vi "ApplyPasswords.vi"() -> ()   [LabVIEW 2009]
panel:
  in  "New Description":string
  in  "Cancel":bool
  in  "Apply":bool
  out "Project Name":string
  in  "Replace Description?":bool=TRUE
  in  "Clear History?":bool=TRUE
  in  "New Password (if empty unlocked)":string
  in  "Old Passwords":string[](array[string])
  out "Progress":dbl(slide) scale=0.0..1.0
  out "Processing VI Name":string
  out "error out":errorcluster
  # "Apply Passwords To Project VIs"
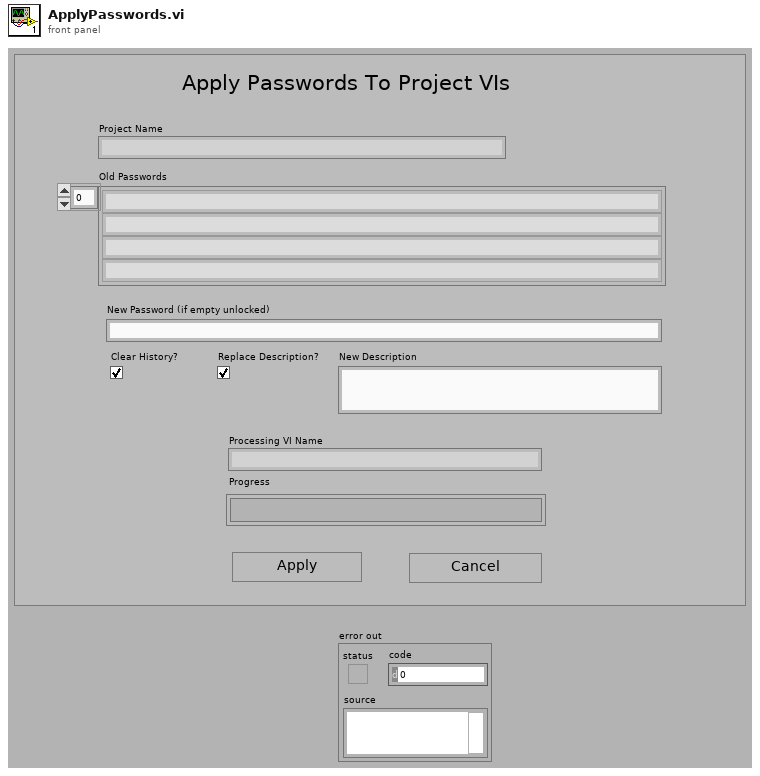
[diagram p1: front panel]
types:
  T1 = enum8{"Enabled", "Disabled", "Disabled and Grayed Out"}
  T2 = enum32{"invalid lock state", "Not Locked", "Locked (No Password)", "Password-protected"}
  T3 = enum32{"invalid VI type", "Standard VI", "Control VI", "Global VI", "Polymorphic VI", "Configuration VI", "SubSystem", "Facade VI", "Method VI", "Statechart Diagram VI"}
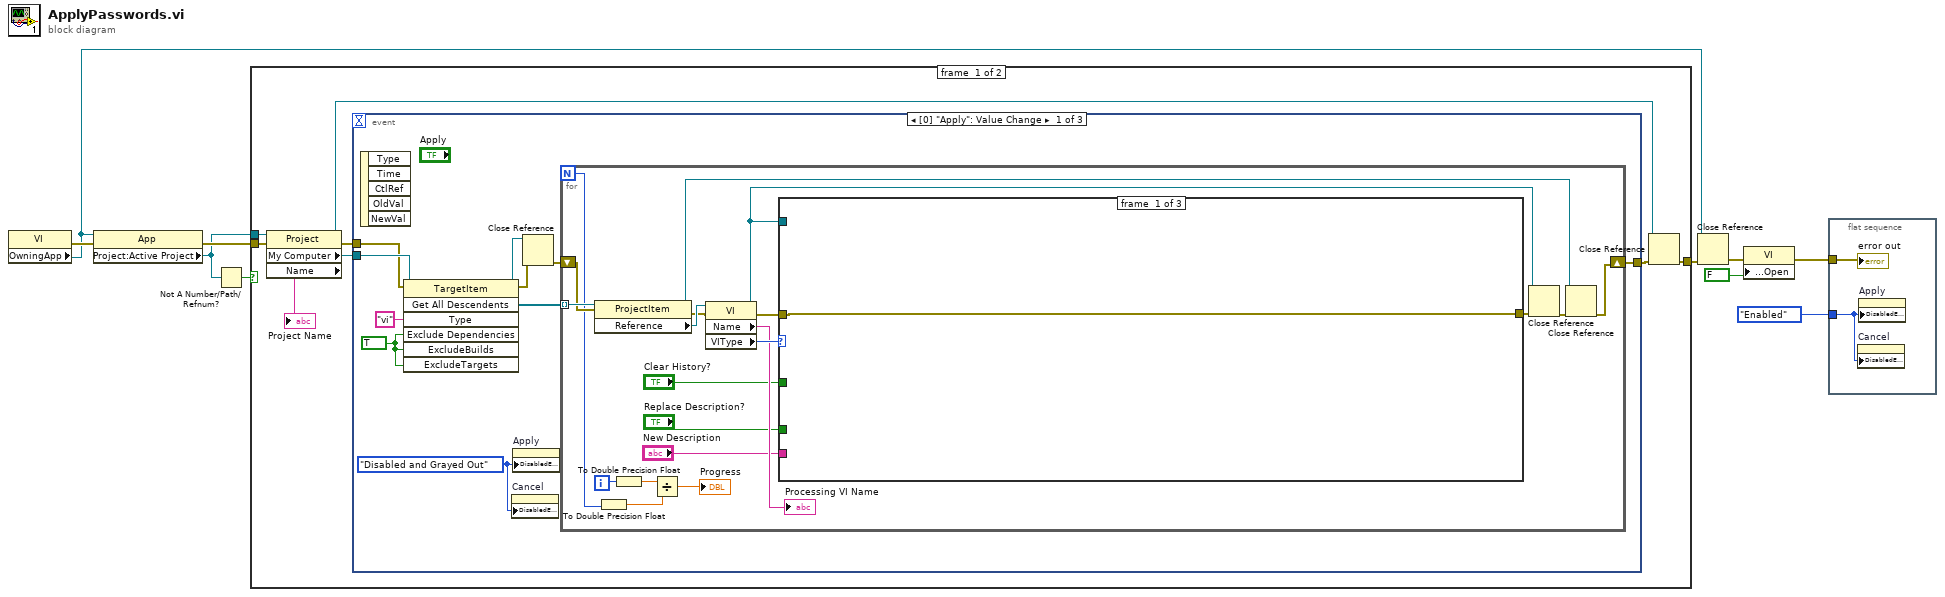
[diagram p0: block diagram]
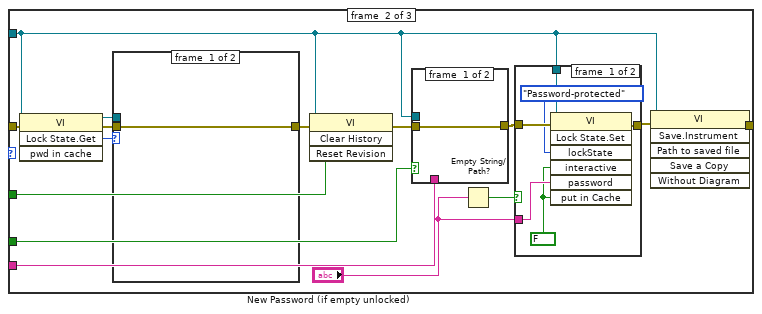
[diagram p2: hidden frame]
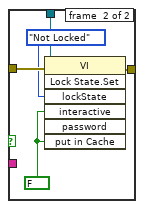
[diagram p3: hidden frame]
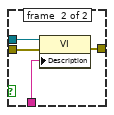
[diagram p4: hidden frame]
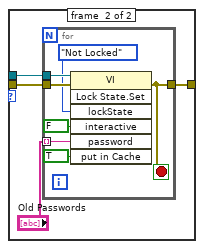
[diagram p5: hidden frame]
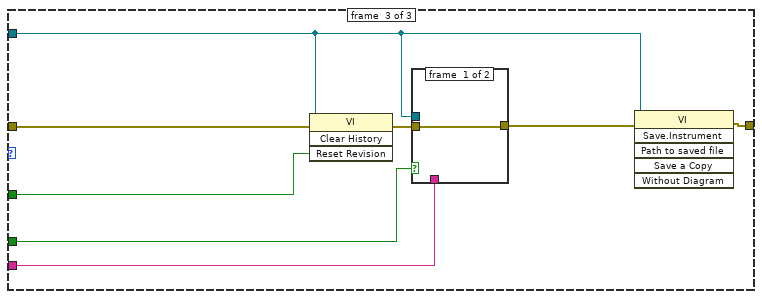
[diagram p6: hidden frame]
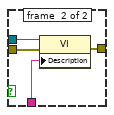
[diagram p7: hidden frame]
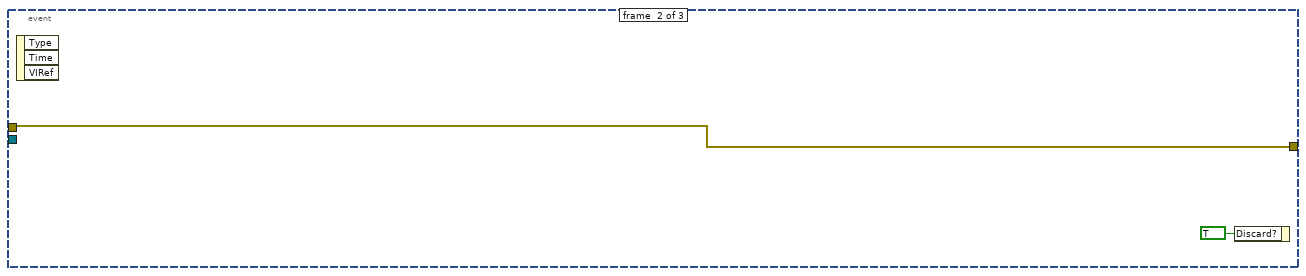
[diagram p8: hidden frame]
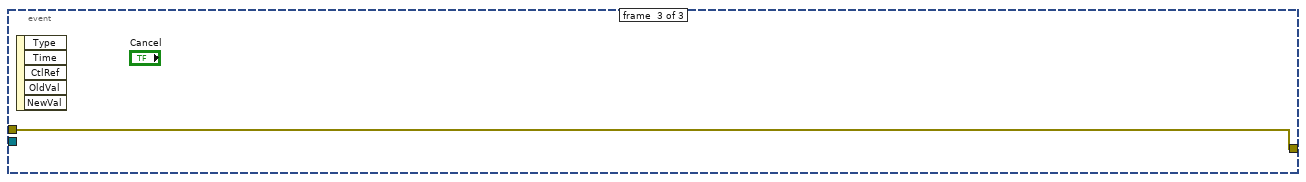
[diagram p9: hidden frame]
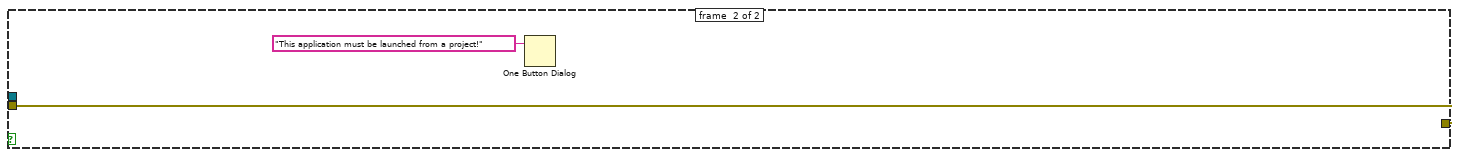
[diagram p10: hidden frame]
diagram:
  n1 = property class="VI"() -> (error out=w10:errorcluster, "OwningApp"=w7:refnum<vi>)  [unwired: 2 in, 1 out]
  n2 = property class="App"(reference=w7, error in=w10) -> (error out=w9:errorcluster, "Project:Active Project"=w6:refnum<vi>)  [unwired: 1 out]
  n3 = Not A Number/Path/Refnum?(number/path/refnum=w6) -> (NaN/Path/Refnum?=w5:bool)
  n4 = case shown="False" w5 {
    tunnel: w9 -> [w18 w110]
    tunnel: [w16 w110] -> w8
    tunnel: w6 -> [w12 _]
    frame #0 {
      n5 = property class="Project"(reference=w12, error in=w18) -> (reference out=w13:refnum<vi>, error out=w15:errorcluster, "My Computer"=w17:refnum<vi>, "Name"=→"Project Name":string)
      n6 = event shown="[0] \"Apply\": Value Change" {
        selector: _ -> [_ _ _]
        dyn-events: _ -> [_ _ _]
        timeout: _ -> [_ _ _]
        tunnel: w17 -> [w28 _ _]
        tunnel: w15 -> [w24 w106 w108]
        tunnel: [w21 w106 w108] -> w14
        event #0 {
          w19 = T1."Disabled and Grayed Out" ("Disabled")
          w27 = TRUE ("ExcludeDependencies")
          n7 = event-data() -> ()  [unwired: 1 in, 5 out]
          n8 = invoke class="TargetItem" method="Get All Descendents"(reference=w28, error in=w24, "Type"="vi", "Exclude Dependencies"=w27, "ExcludeBuilds"=w27, "ExcludeTargets"=w27) -> (reference out=w23:refnum<vi>, error out=w25:errorcluster, "All Descendents"=w26:refnum<vi>[])  [unwired: 1 in, 4 out]
          n9 = property on="Cancel" class="Bool"("DisabledEnum"=w19) -> ()  [unwired: 2 in, 2 out]
          n10 = property on="Apply" class="Bool"("DisabledEnum"=w19) -> ()  [unwired: 2 in, 2 out]
          n11 = Close Reference(reference=w23, error in (no error)=w25) -> (error out=w22:errorcluster)
          n12 = for {
            N -> [w38]
            tunnel: w26 -> [w48] mode=indexing
            shift-right: [w46] -> w21
            shift-left: w22 -> [w47]
            i -> [w39]
            n13 = property class="ProjectItem"(reference=w48, error in=w47) -> (reference out=w45:refnum<vi>, error out=w43:errorcluster, "Reference"=w44:refnum<vi>)
            n14 = To Double Precision Float(number=w38) -> (double precision float=w36:dbl)
            n15 = To Double Precision Float(number=w39) -> (double precision float=w37:dbl)
            n16 = Divide(x=w37, y=w36) -> (x/y=→"Progress":dbl)
            n17 = property class="VI"(reference=w44, error in=w43) -> (reference out=w34:refnum<vi>, error out=w40:errorcluster, "Name"=→"Processing VI Name":string, "VIType"=w41:T3)
            n18 = case shown="\"Control VI\"" w41 {
              tunnel: w40 -> [w49 w64 w97]
              tunnel: w34 -> [_ w53 w98]
              tunnel: [w49 w55 w99] -> w33
              tunnel: "Clear History?" -> [_ w52 w96]
              tunnel: "Replace Description?" -> [_ w51 w95]
              tunnel: "New Description" -> [_ w50 w94]
              frame #0 {
              }
              frame #1 {
                n19 = invoke class="VI" method="Lock State.Get"(reference=w53, error in=w64) -> (reference out=w61:refnum<vi>, error out=w62:errorcluster, "Get Lock State"=w63:T2)  [unwired: 2 in, 1 out]
                n20 = case shown="\"Locked (No Password)\", \"Password-protected\"" w63 {
                  tunnel: w62 -> [w81 w85]
                  tunnel: w61 -> [_ w84]
                  tunnel: [w81 w82] -> w60
                  frame #0 {
                  }
                  frame #1 {
                    n21 = for {
                      tunnel: w84 -> [w92]
                      tunnel: "Old Passwords" -> [w90] mode=indexing
                      tunnel: w85 -> [w91]
                      tunnel: [w89] -> w82
                      stop <- w89 stop-if-true
                      n22 = invoke class="VI" method="Lock State.Set"(reference=w92, error in=w91, "lockState"=T2."Not Locked" ("Lock State"), "interactive"=FALSE ("Interactive"), "password"=w90, "put in Cache"=TRUE ("Put in Cache")) -> (error out=w89:errorcluster)  [unwired: 1 in, 6 out]
                    }
                  }
                }
                n23 = invoke class="VI" method="Clear History"(reference=w53, error in=w60, "Reset Revision"=w52) -> (error out=w59:errorcluster)  [unwired: 1 in, 3 out]
                n24 = case shown="True" w51 {
                  tunnel: w59 -> [w76 w80]
                  tunnel: w53 -> [_ w79]
                  tunnel: [w76 w78] -> w58
                  tunnel: w50 -> [_ w77]
                  frame #0 {
                  }
                  frame #1 {
                    n25 = property class="VI"(reference=w79, error in=w80, "Description"=w77) -> (error out=w78:errorcluster)  [unwired: 1 out]
                  }
                }
                n26 = Empty String/Path?(string/path="New Password (if empty unlocked)") -> (empty?=w57:bool)
                n27 = case shown="True" w57 {
                  tunnel: w58 -> [w70 w75]
                  tunnel: [w69 w74] -> w54
                  tunnel: w53 -> [w68 w73]
                  tunnel: "New Password (if empty unlocked)" -> [w67 _]
                  frame #0 {
                    w65 = FALSE
                    n28 = invoke class="VI" method="Lock State.Set"(reference=w68, error in=w70, "lockState"=T2."Password-protected" ("Lock State"), "interactive"=w65, "password"=w67, "put in Cache"=w65) -> (error out=w69:errorcluster)  [unwired: 1 in, 6 out]
                  }
                  frame #1 {
                    w71 = FALSE
                    n29 = invoke class="VI" method="Lock State.Set"(reference=w73, error in=w75, "lockState"=T2."Not Locked" ("Lock State"), "interactive"=w71, "put in Cache"=w71) -> (error out=w74:errorcluster)  [unwired: 2 in, 6 out]
                  }
                }
                n30 = invoke class="VI" method="Save.Instrument"(reference=w53, error in=w54) -> (error out=w55:errorcluster)  [unwired: 4 in, 5 out]
              }
              frame #2 {
                n31 = invoke class="VI" method="Clear History"(reference=w98, error in=w97, "Reset Revision"=w96) -> (error out=w100:errorcluster)  [unwired: 1 in, 3 out]
                n32 = case shown="True" w95 {
                  tunnel: w100 -> [w101 w105]
                  tunnel: w98 -> [_ w104]
                  tunnel: [w101 w103] -> w93
                  tunnel: w94 -> [_ w102]
                  frame #0 {
                  }
                  frame #1 {
                    n33 = property class="VI"(reference=w104, error in=w105, "Description"=w102) -> (error out=w103:errorcluster)  [unwired: 1 out]
                  }
                }
                n34 = invoke class="VI" method="Save.Instrument"(reference=w98, error in=w93) -> (error out=w99:errorcluster)  [unwired: 4 in, 5 out]
              }
            }
            n35 = Close Reference(reference=w34, error in (no error)=w33) -> (error out=w42:errorcluster)
            n36 = Close Reference(reference=w45, error in (no error)=w42) -> (error out=w46:errorcluster)
          }
        }
        event #1 {
          n37 = event-data() -> ()  [unwired: 1 in, 3 out]
          n38 = event-data("Discard?"=TRUE) -> ()  [unwired: 1 in, 1 out]
        }
        event #2 {
          n39 = event-data() -> ()  [unwired: 1 in, 5 out]
        }
      }
      n40 = Close Reference(reference=w13, error in (no error)=w14) -> (error out=w16:errorcluster)
    }
    frame #1 {
      n41 = One Button Dialog(message="This application must be launched from a project!") -> ()  [unwired: 1 in, 1 out]
    }
  }
  n42 = Close Reference(reference=w7, error in (no error)=w8) -> (error out=w4:errorcluster)
  n43 = property class="VI"(error in=w4, "Front Panel.Open"=FALSE ("Front Panel Window:Open")) -> (error out=w3:errorcluster)  [unwired: 1 in, 1 out]
  n44 = flat-sequence {
    tunnel: w3 -> [w112]
    tunnel: T1."Enabled" ("Disabled") -> [w111]
    frame #0 {
      n45 = property on="Cancel" class="Bool"("DisabledEnum"=w111) -> ()  [unwired: 2 in, 2 out]
      n46 = property on="Apply" class="Bool"("DisabledEnum"=w111) -> ()  [unwired: 2 in, 2 out]
      "error out" <- w112
    }
  }
